vi "Projection Matrix.vi"   [LabVIEW 2022 SP3, in "3D Tests.lvclass"]
uses:
  3D Tests.lvclass
  Libraries/Raster/Screen Dimensions.ctl
  Libraries/3D/Camera.ctl
  <vilib>/addons/_JKI Toolkits/Caraya/classes/Assert/Assert Equal Value and Type_Variant.vi
  <vilib>/addons/_JKI Toolkits/Caraya/classes/Test/Test.lvclass
  Libraries/3D/3D.lvlib
  Libraries/Raster/Raster.lvlib
  <vilib>/addons/_JKI Toolkits/Caraya/classes/Assert/Assert.lvclass
types:
  T1 = typedef "3D.lvlib/Camera.ctl" = cluster{"Field Of View":sgl, "Near Plane":sgl, "Far Plane":sgl}
  T2 = typedef "Raster.lvlib/Screen Dimensions.ctl" = cluster{"Width":u32, "Height":u32}
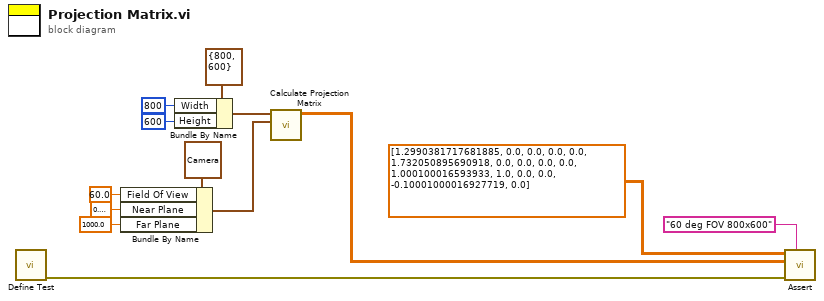
[diagram p0: block diagram]
diagram:
  n1 = call <vilib>:"Define Test.vi"() -> ("error out"=w4:errorcluster)  [unwired: 11 in]
  n2 = Bundle By Name(cluster=T1 {"Field Of View"=60.0, "Near Plane"=0.1, "Far Plane"=1000.0} ("Camera"), "Field Of View"=sgl 60.0, "Near Plane"=sgl 0.1, "Far Plane"=sgl 1000.0) -> (w12:T1)
  n3 = Bundle By Name(cluster=T2 {"Width"=800, "Height"=600} ("Screen Dimensions"), "Width"=u32 800, "Height"=u32 600) -> (w7:T2)
  n4 = call "Calculate Projection Matrix.vi"("Camera"=w12, "Screen Dimensions"=w7) -> ("Projection Matrix"=w2:sgl[][])  [unwired: 9 in]
  n5 = call-poly <vilib>:"Assert.vi"("Label"="60 deg FOV 800x600", "error in (no error)"=w4, "Y"=w2, "X"=sgl[][] [[1.2990382, 0.0, 0.0, 0.0], [0.0, 1.7320509, 0.0, 0.0], [0.0, 0.0, 1.0001, 1.0], [0.0, 0.0, -0.10001, 0.0]] ("Projection Matrix")) -> ()  [unwired: 7 in, 1 out]
